vi "Send Task Outputs.vi"(4 "Status":string="Built", 6 "Build Specification Version":T1, 8 "error in (no error)":errorcluster, 9 "Generated files":path[](array[path]), 10 "Task":refnum<class "Task.lvclass">, 11 "BuildWorker in":refnum<class "BuildWorker.lvclass">) -> (0 "error out":errorcluster, 3 "BuildWorker out":refnum<class "BuildWorker.lvclass">)   [LabVIEW 2017, in "BuildWorker.lvlib" / "BuildWorker.lvclass"]
uses:
  BuildWorker.lvclass
  Classes/Task Interface/Task/Task.lvclass
  <vilib>/AppBuilder/AB_API_Simple/Build Specification Version.ctl
  BuildWorker.lvclass/BuildWorker.ctl
  Classes/Task Interface/Task/Task.lvclass/Task.ctl
  Communication/WebSocket Client/WebSocket Client Messages/Send Message Msg/Send Message Msg.lvclass/Send Message Msg.ctl
  <vilib>/ActorFramework/Message Enqueuer/Message Enqueuer.lvclass/Message Enqueuer.ctl
  Classes/Task Interface/Task/Get Name.vi
  <vilib>/ActorFramework/Message Enqueuer/Enqueue.vi
  Communication/WebSocket Client/WebSocket Client Messages/Send Message Msg/Send Message Msg.lvclass
  C:/Program Files (x86)/National Instruments/LabVIEW 2017/vi.lib/ActorFramework/Message/Message.lvclass
  <vilib>/ActorFramework/Message Priority Queue/Priority Enqueue.vi
  Classes/Message Interface/Task Outputs/Task Outputs.lvclass
  <vilib>/AppBuilder/AB_API_Simple/NI_App_Builder_API.lvlib
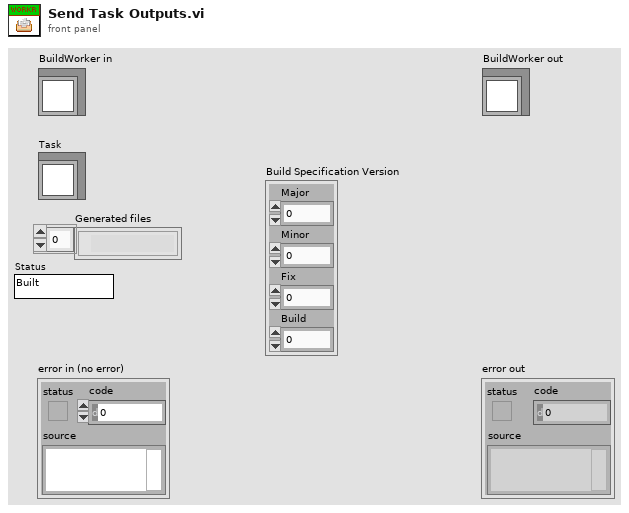
[diagram p1: front panel]
types:
  T1 = typedef "NI_App_Builder_API.lvlib/Build Specification Version.ctl" = cluster{"Major":u16, "Minor":u16, "Fix":u16, "Build":u16}
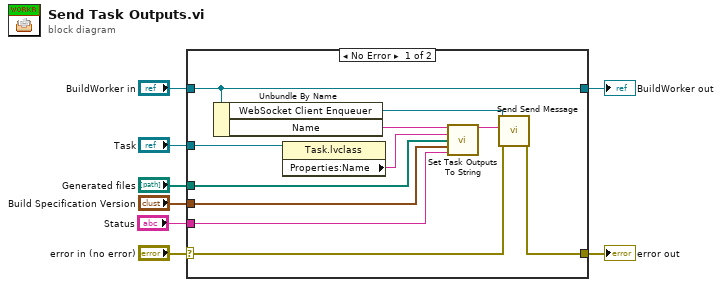
[diagram p0: block diagram]
diagram:
  n1 = case shown="No Error" "error in (no error)" {
    selector: "error in (no error)" -> [w16 w21]
    tunnel: [w15 w21] -> w7
    tunnel: [w19 w20] -> w5
    tunnel: "BuildWorker in" -> [w19 w20]
    tunnel: "Task" -> [w18 _]
    tunnel: "Generated files" -> [w12 _]
    tunnel: "Build Specification Version" -> [w11 _]
    tunnel: "Status" -> [w10 _]
    frame No Error {
      n2 = Unbundle By Name(w19) -> ("WebSocket Client Enqueuer"=w17:refnum<class "Message Enqueuer.lvclass">, "Name"=w14:string)
      n3 = property class="Task.lvclass"(reference=w18) -> ("Properties:Name"=w13:string)  [unwired: 1 in, 2 out]
      n4 = call "Set Task Outputs To String.vi"("Sender"=w14, "Item Name"=w13, "Generated Files"=w12, "Build Specification Version"=w11, "Status"=w10) -> ("data string"=w9:string)  [unwired: 10 in]
      n5 = call "Send Send Message.vi"("error in (no error)"=w16, "Message"=w9, "Message Enqueuer in"=w17) -> ("error out"=w15:errorcluster)  [unwired: 7 in, 1 out]
    }
    frame Error {
    }
  }
  "error out" <- w7
  "BuildWorker out" <- w5
